vi "Write New Data Msg.vi"(10 "Test_Nested.lvlib:New Data Msg.lvclass":refnum<class "New Data Msg.lvclass">, 11 "Test_Nested in":refnum<class "Test_Nested.lvclass">) -> (3 "Test_Nested out":refnum<class "Test_Nested.lvclass">)   [LabVIEW 2025, in "Test_Nested.lvlib" / "Test_Nested.lvclass"]
uses:
  Test_Nested.lvclass
  Test_Nested Messages/New Data Msg/New Data Msg.lvclass
  Test_Nested.lvclass/Test_Nested.ctl
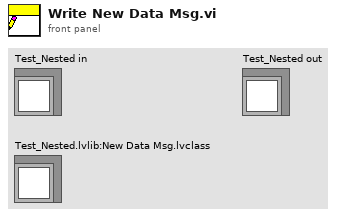
[diagram p1: front panel]
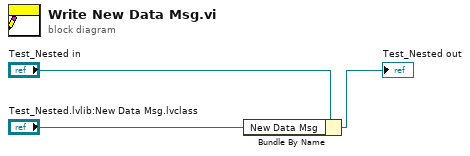
[diagram p0: block diagram]
diagram:
  n1 = Bundle By Name(cluster="Test_Nested in", "New Data Msg"="Test_Nested.lvlib:New Data Msg.lvclass") -> (→"Test_Nested out":refnum<class "Test_Nested.lvclass">)
